vi "subLogPPLReplace.vi"(9 "Log info":T1, 11 "Byte Stream File in":refnum<file>) -> (0 "error out":errorcluster, 3 "refnum out":refnum<file>)   [LabVIEW 2019, in "SolutionBuilder.lvlib" / "BuildManager.lvclass"]
uses:
  BuildManager.lvclass
  LogInfo.ctl
  SolutionBuilder.lvlib
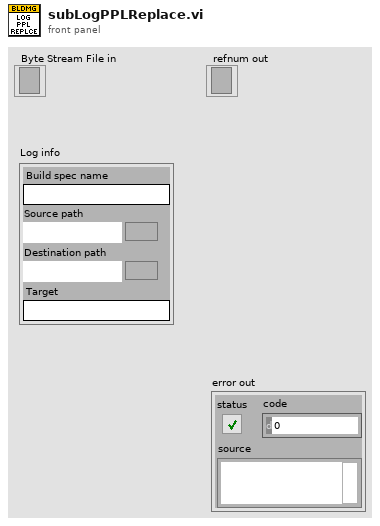
[diagram p1: front panel]
types:
  T1 = typedef "SolutionBuilder.lvlib/BuildManager.lvclass/LogInfo.ctl" = cluster{"Build spec name":string, "Source path":path, "Destination path":path, "Target":string}
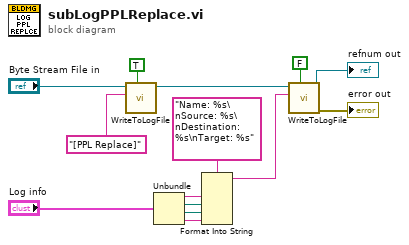
[diagram p0: block diagram]
diagram:
  n1 = call "WriteToLogFile.vi"("Prepend timestamp"=TRUE, "Log entry"="[PPL Replace]" ("format string"), "Byte Stream File in"="Byte Stream File in") -> ("refnum out"=w4:refnum<file>)  [unwired: 7 in, 1 out]
  n2 = Unbundle("Log info") -> ("Build spec name"=w12:string, "Source path"=w11:path, "Destination path"=w9:path, "Target"=w10:string)
  n3 = Format Into String(format string="Name: %s\nSource: %s\nDestination: %s\nTarget: %s", w12, w11, w9, w10) -> (resulting string=w3:string)  [unwired: 2 in, 1 out]
  n4 = call "WriteToLogFile.vi"("Prepend timestamp"=FALSE, "Log entry"=w3, "Byte Stream File in"=w4) -> ("error out"=→"error out":errorcluster, "refnum out"=→"refnum out":refnum<file>)  [unwired: 7 in]
